vi "CODMn测量流程.vi"(11 "控制命令":T1(ring)) -> ()   [LabVIEW 2016, in "斯坦道CODMn.lvlib"]
panel:
  out "start":timestamp
  out "补测":bool
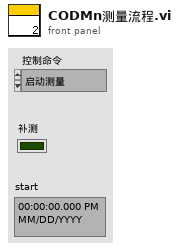
[diagram p1: front panel]
types:
  T1 = enum16{"启动测量", "标样核查", "零点核查", "跨度核查", "空白测试", "平行样测试", "加标回收", "空白校准", "标样校准", "初始化（清洗）", "停止测试", "仪器重启", "校时", "模式设置", "测量间隔设置"}
  T2 = cluster{"测量模式":enum16{"水样测量", "标样核查", "零点核查", "跨度核查", "空白测试", "加标回收", "平行样", "校零", "校标"}}
  T3 = enum16{"空闲", "水样测试", "标样核查", "零点核查", "跨度核查", "空白测试", "平行样测试", "质控样", "空白校准", "标样校准", "加标回收"}
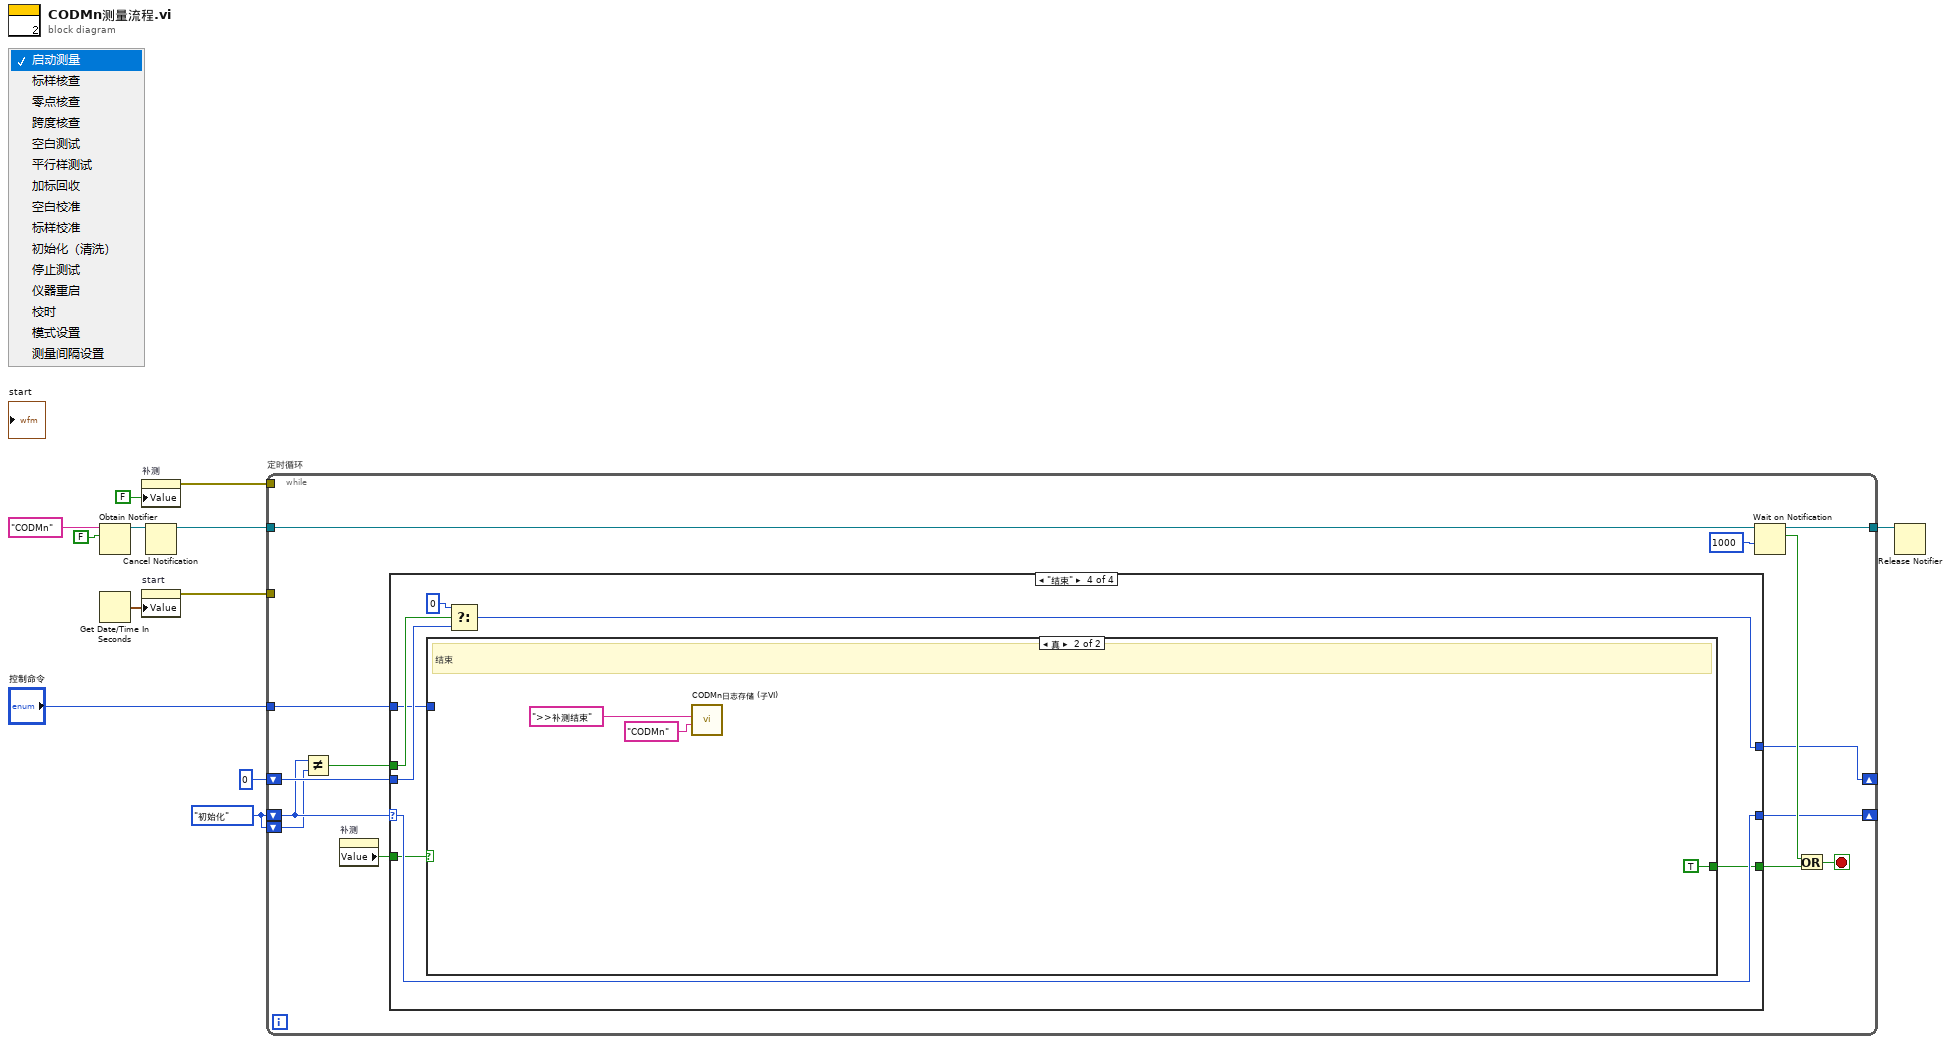
[diagram p0: block diagram]
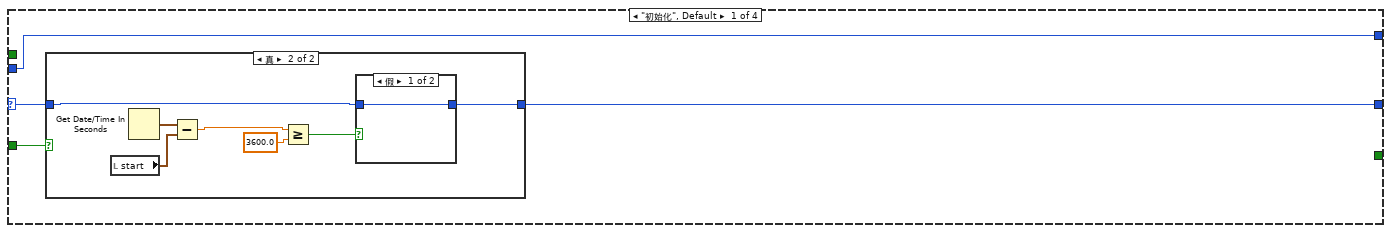
[diagram p2: hidden frame]
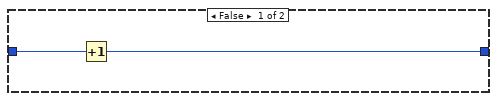
[diagram p3: hidden frame]
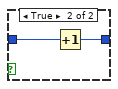
[diagram p4: hidden frame]
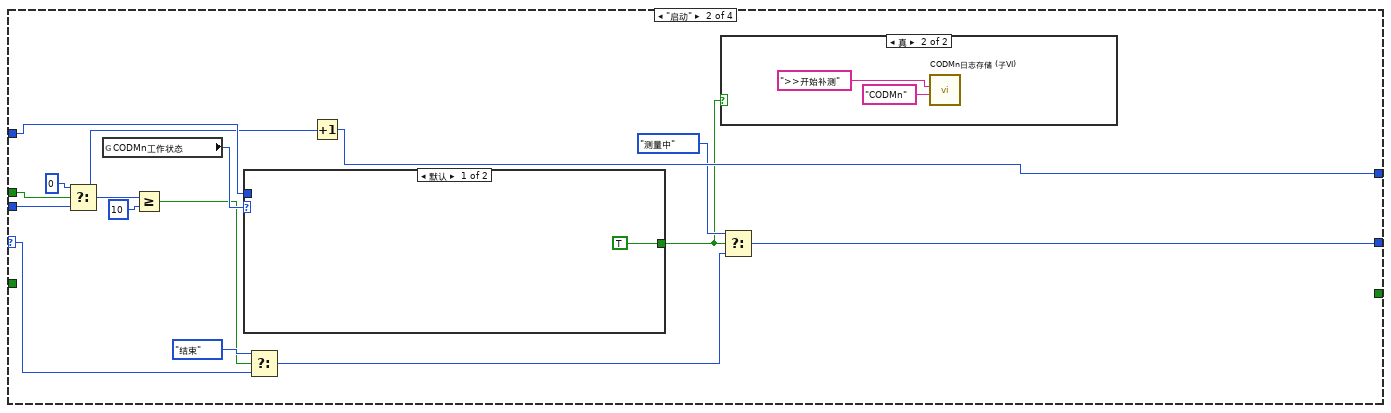
[diagram p5: hidden frame]
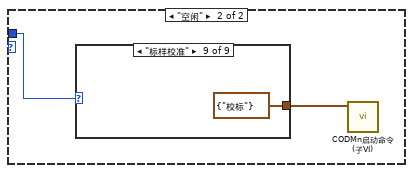
[diagram p7: hidden frame]
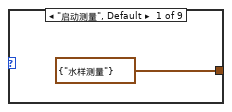
[diagram p8: hidden frame]
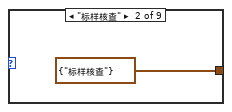
[diagram p9: hidden frame]
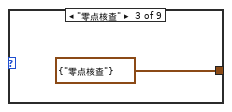
[diagram p10: hidden frame]
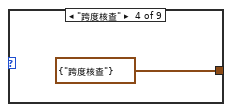
[diagram p11: hidden frame]
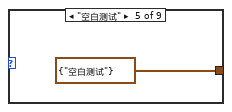
[diagram p12: hidden frame]
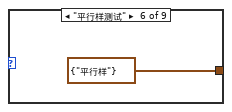
[diagram p13: hidden frame]
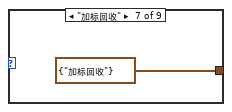
[diagram p14: hidden frame]
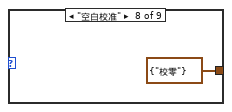
[diagram p15: hidden frame]
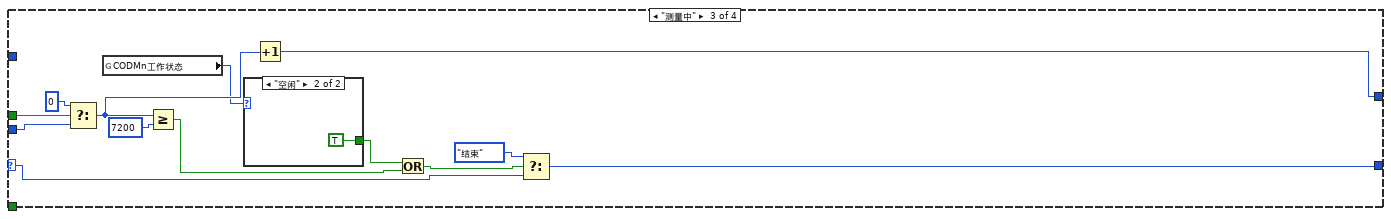
[diagram p16: hidden frame]
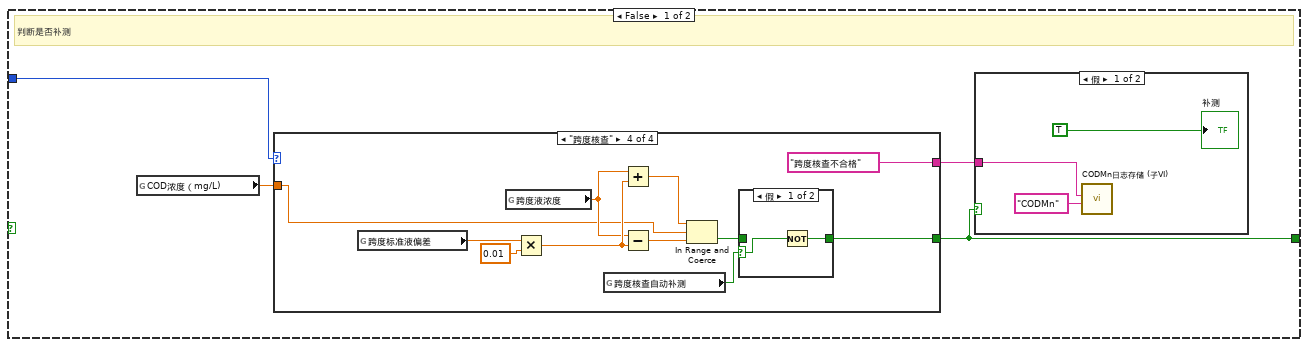
[diagram p18: hidden frame]
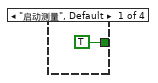
[diagram p20: hidden frame]
diagram:
  w5 = enum16{"初始化", "启动", "测量中", "结束"}."初始化"
  n1 = Obtain Notifier(name (unnamed)="CODMn" ("名称（未命名）"), notification data type=FALSE) -> (notifier out=w10:refnum<notifier>)  [unwired: 2 in, 2 out]
  n2 = Get Date/Time In Seconds() -> (seconds since 1Jan1904=w4:timestamp)
  n3 = property on="补测" class="Bool (严格)"("Value"=FALSE ("补测")) -> (error out=w2:errorcluster)  [unwired: 2 in, 1 out]
  n4 = property on="start" class="AbsTime (严格)"("Value"=w4) -> (error out=w1:errorcluster)  [unwired: 2 in, 1 out]
  n5 = Cancel Notification(0:w10) -> (8:w9:refnum<notifier>)  [unwired: 1 in, 2 out]
  n6 = while "定时循环" {
    tunnel: w9 -> [w26]
    tunnel: "控制命令" -> [w22]
    shift-right: [w21] -> _
    shift-left: w5 -> [w16]
    shift-right: [w19] -> _
    shift-left: 0 -> [w20]
    tunnel: [w17] -> w7
    shift-left: w5 -> [w15]
    tunnel: w2 -> [_]
    tunnel: w1 -> [_]
    stop <- w23 stop-if-true
    n7 = Not Equal?(x=w16, y=w15) -> (x != y?=w14:bool)
    n8 = property on="补测" class="Bool (严格)"() -> ("Value"=w13:bool)  [unwired: 2 in, 2 out]
    n9 = case shown="\"结束\"" w16 {
      selector: w16 -> [w30 w51 w72 w93]
      tunnel: w22 -> [_ w57 _ w87]
      tunnel: [w29 w46 w75 w93] -> w21
      tunnel: w20 -> [w28 w55 w83 w91]
      tunnel: [w28 w54 w82 w90] -> w19
      tunnel: [_ _ _ w86] -> w18
      tunnel: w14 -> [_ w48 w77 w89]
      tunnel: w13 -> [w27 _ _ w88]
      frame "初始化", Default {
        n10 = case shown="真" w27 {
          tunnel: w30 -> [w32 w34]
          tunnel: [w31 w33] -> w29
          frame False {
            n11 = Increment(x=w32) -> (x+1=w31:enum16{"初始化", "启动", "测量中", "结束"})
          }
          frame True {
            n12 = local read "start"() -> (w38:timestamp)
            n13 = Get Date/Time In Seconds() -> (seconds since 1Jan1904=w39:timestamp)
            n14 = Subtract(x=w39, y=w38) -> (x-y=w36:dbl)
            n15 = Greater Or Equal?(x=w36, y=3600.0) -> (x >= y?=w35:bool)
            n16 = case shown="假" w35 {
              tunnel: w34 -> [w40 w42]
              tunnel: [w40 w41] -> w33
              frame False {
              }
              frame True {
                n17 = Increment(x=w42) -> (x+1=w41:enum16{"初始化", "启动", "测量中", "结束"})
              }
            }
          }
        }
      }
      frame "启动" {
        n18 = Select(t=0, s=w48, f=w55) -> (s? t:f=w53:i32)
        n19 = global read "COD测量模式全局.vi" "CODMn工作状态"() -> (w49:T3)
        n20 = Greater Or Equal?(x=w53, y=10) -> (x >= y?=w44:bool)
        n21 = case shown="默认" w49 {
          tunnel: w57 -> [_ w62]
          tunnel: [TRUE _] -> w43
          frame Default {
          }
          frame "空闲" {
            n22 = case shown="\"标样校准\"" w62 {
              tunnel: [T2 {"测量模式"=enum."水样测量"} ("启动测量模式") T2 {"测量模式"=enum."标样核查"} ("启动测量模式") T2 {"测量模式"=enum."零点核查"} ("启动测量模式") T2 {"测量模式"=enum."跨度核查"} ("启动测量模式") T2 {"测量模式"=enum."空白测试"} ("启动测量模式") T2 {"测量模式"=enum."平行样"} ("启动测量模式") T2 {"测量模式"=enum."加标回收"} ("启动测量模式") T2 {"测量模式"=enum."校零"} ("启动测量模式") T2 {"测量模式"=enum."校标"} ("启动测量模式")] -> w61
              frame "启动测量", Default {
              }
              frame "标样核查" {
              }
              frame "零点核查" {
              }
              frame "跨度核查" {
              }
              frame "空白测试" {
              }
              frame "平行样测试" {
              }
              frame "加标回收" {
              }
              frame "空白校准" {
              }
              frame "标样校准" {
              }
            }
            n23 = call "CODMn启动命令 (子VI).vi"("启动测量模式"=w61) -> ()  [unwired: 11 in]
          }
        }
        n24 = Select(t=enum16{"初始化", "启动", "测量中", "结束"}."结束", s=w44, f=w51) -> (s? t:f=w47:enum16{"初始化", "启动", "测量中", "结束"})
        n25 = Increment(x=w53) -> (x+1=w54:i32)
        n26 = case shown="真" w43 {
          frame False {
          }
          frame True {
            n27 = call "CODMn日志存储 (子VI).vi"("参数"="CODMn" ("设备"), "日志信息"=">>开始补测") -> ()  [unwired: 10 in]
          }
        }
        n28 = Select(t=enum16{"初始化", "启动", "测量中", "结束"}."测量中", s=w43, f=w47) -> (s? t:f=w46:enum16{"初始化", "启动", "测量中", "结束"})
      }
      frame "测量中" {
        n29 = Select(t=0, s=w77, f=w83) -> (s? t:f=w81:i32)
        n30 = global read "COD测量模式全局.vi" "CODMn工作状态"() -> (w78:T3)
        n31 = Greater Or Equal?(x=w81, y=7200) -> (x >= y?=w76:bool)
        n32 = case shown="\"空闲\"" w78 {
          tunnel: [_ TRUE] -> w73
          frame Default {
          }
          frame "空闲" {
          }
        }
        n33 = Increment(x=w81) -> (x+1=w82:i32)
        n34 = Or(x=w73, y=w76) -> (x .or. y?=w74:bool)
        n35 = Select(t=enum16{"初始化", "启动", "测量中", "结束"}."结束", s=w74, f=w72) -> (s? t:f=w75:enum16{"初始化", "启动", "测量中", "结束"})
      }
      frame "结束" {
        n36 = case shown="真" w88 {
          tunnel: w87 -> [w97 _]
          tunnel: [w94 TRUE] -> w86
          frame False {
            # "判断是否补测"
            n37 = global read "COD浓度全局变量.vi" "COD浓度（mg/L)"() -> (w96:dbl)
            n38 = case shown="\"跨度核查\"" w97 {
              tunnel: w96 -> [_ w107 w121 w135]
              tunnel: [_ "标样核查不合格" ("日志信息") "零点核查不合格" ("日志信息") "跨度核查不合格" ("日志信息")] -> w95
              tunnel: [TRUE w102 w116 w130] -> w94
              frame "启动测量", Default {
              }
              frame "标样核查" {
                n39 = global read "CODMn断电保存全局变量.vi" "标准液标准偏差"() -> (w106:dbl)
                n40 = Multiply(x=w106, y=0.01) -> (x*y=w111:dbl)
                n41 = global read "CODMn断电保存全局变量.vi" "标样浓度"() -> (w108:dbl)
                n42 = global read "CODMn断电保存全局变量.vi" "标样核查自动补测"() -> (w105:bool)
                n43 = Add(x=w108, y=w111) -> (x+y=w110:dbl)
                n44 = Subtract(x=w108, y=w111) -> (x-y=w109:dbl)
                n45 = In Range and Coerce(upper limit=w110, x=w107, lower limit=w109) -> (In Range?=w104:bool)  [unwired: 1 out]
                n46 = case shown="假" w105 {
                  selector: w105 -> [w114 _]
                  tunnel: w104 -> [_ w115]
                  tunnel: [w113 w115] -> w102
                  frame False {
                    n47 = Not(x=w114) -> (.not. x?=w113:bool)
                  }
                  frame True {
                  }
                }
              }
              frame "零点核查" {
                n48 = global read "CODMn断电保存全局变量.vi" "零点标准液偏差"() -> (w120:dbl)
                n49 = global read "CODMn断电保存全局变量.vi" "零点核查浓度"() -> (w122:dbl)
                n50 = Multiply(x=w120, y=1.0) -> (x*y=w125:dbl)
                n51 = global read "CODMn断电保存全局变量.vi" "零点核查自动补测"() -> (w119:bool)
                n52 = Add(x=w122, y=w125) -> (x+y=w124:dbl)
                n53 = Subtract(x=w122, y=w125) -> (x-y=w123:dbl)
                n54 = In Range and Coerce(upper limit=w124, x=w121, lower limit=w123) -> (In Range?=w118:bool)  [unwired: 1 out]
                n55 = case shown="假" w119 {
                  selector: w119 -> [w128 _]
                  tunnel: w118 -> [_ w129]
                  tunnel: [w127 w129] -> w116
                  frame False {
                    n56 = Not(x=w128) -> (.not. x?=w127:bool)
                  }
                  frame True {
                  }
                }
              }
              frame "跨度核查" {
                n57 = global read "CODMn断电保存全局变量.vi" "跨度标准液偏差"() -> (w134:dbl)
                n58 = global read "CODMn断电保存全局变量.vi" "跨度液浓度"() -> (w136:dbl)
                n59 = Multiply(x=w134, y=0.01) -> (x*y=w139:dbl)
                n60 = global read "CODMn断电保存全局变量.vi" "跨度核查自动补测"() -> (w133:bool)
                n61 = Add(x=w136, y=w139) -> (x+y=w138:dbl)
                n62 = Subtract(x=w136, y=w139) -> (x-y=w137:dbl)
                n63 = In Range and Coerce(upper limit=w138, x=w135, lower limit=w137) -> (In Range?=w132:bool)  [unwired: 1 out]
                n64 = case shown="假" w133 {
                  selector: w133 -> [w142 _]
                  tunnel: w132 -> [_ w143]
                  tunnel: [w141 w143] -> w130
                  frame False {
                    n65 = Not(x=w142) -> (.not. x?=w141:bool)
                  }
                  frame True {
                  }
                }
              }
            }
            n66 = case shown="假" w94 {
              tunnel: w95 -> [w99 _]
              frame False {
                n67 = call "CODMn日志存储 (子VI).vi"("参数"="CODMn" ("设备"), "日志信息"=w99) -> ()  [unwired: 10 in]
                "补测" <- TRUE ("补测")
              }
              frame True {
              }
            }
          }
          frame True {
            # "结束"
            n68 = call "CODMn日志存储 (子VI).vi"("参数"="CODMn" ("设备"), "日志信息"=">>补测结束") -> ()  [unwired: 10 in]
          }
        }
        n69 = Select(t=0, s=w89, f=w91) -> (s? t:f=w90:i32)
      }
    }
    n70 = Wait on Notification(notifier=w26, timeout in ms (-1)=1000 ("超时毫秒(-1)")) -> (notifier out=w17:refnum<notifier>, notification=w24:bool)  [unwired: 2 in, 2 out]
    n71 = Or(x=w24, y=w18) -> (x .or. y?=w23:bool)
  }
  n72 = Release Notifier(notifier=w7) -> ()  [unwired: 2 in, 3 out]
